vi "get data string.vi"(6 "dataToGet":i32, 9 "read buffer in":string, 10 "unsigned byte array":u8[](array[numeric]), 11 "startIdx":u8) -> (2 "read buffer out":string, 3 "lastIdx":u8)   [LabVIEW 2014, in "HPCNC.lvlib"]
uses:
  HPCNC.lvlib
  GetCncPosition.dll
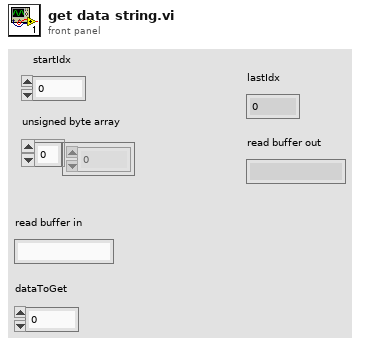
[diagram p1: front panel]
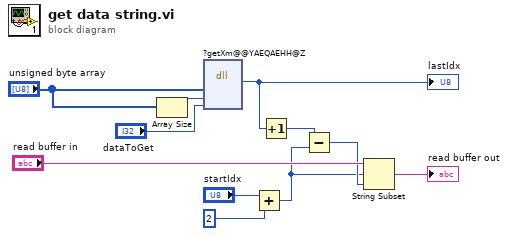
[diagram p0: block diagram]
diagram:
  n1 = Array Size(array="unsigned byte array") -> (size(s)=w6:i32)
  n2 = dll-call lib="D:/Workspace/Giang/Labview/Minigantry With FS/SubVIs/GetCncPosition.dll" fn="?getXm@@YAEQAEHH@Z" label="dataindex"("arrayI"="unsigned byte array", "size"=w6, "dataToGet"="dataToGet") -> ("return type"=w7:u8)  [unwired: 6 in, 2 out]
  "lastIdx" <- w7
  n3 = Add(x="startIdx", y=u8 2) -> (x+y=w1:u8)
  n4 = Increment(x=w7) -> (x+1=w8:u8)
  n5 = Subtract(x=w8, y=w1) -> (x-y=w10:u8)
  n6 = String Subset(string="read buffer in", offset (0)=w1, length (rest)=w10) -> (substring=→"read buffer out":string)
